vi "23_Roots of Eqn using Case.vi"() -> ()   [LabVIEW 2022 SP3]
panel:
  out "Inference:":string
  out "Root 2":dbl
  out "Root 1":dbl
  in  "C":dbl
  in  "B":dbl
  in  "A":dbl
  # "Develop a HMI to find the roots of an equation and categorize\n whether its Real&Equal or Real&Unequal using Case structure"
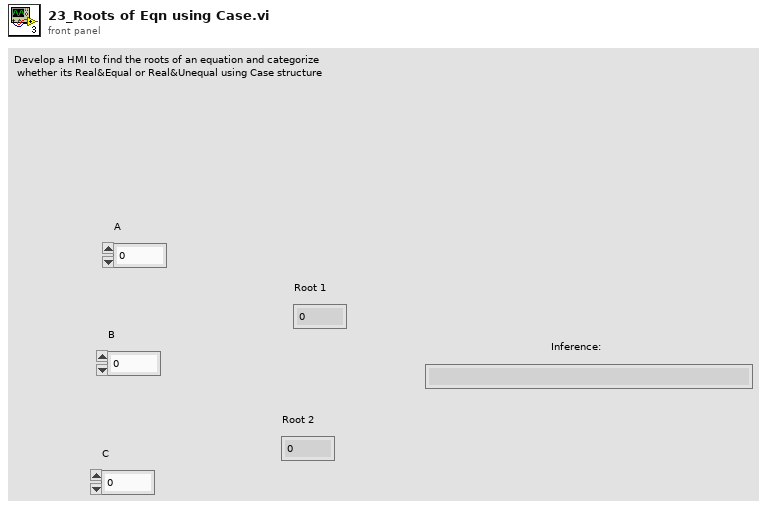
[diagram p1: front panel]
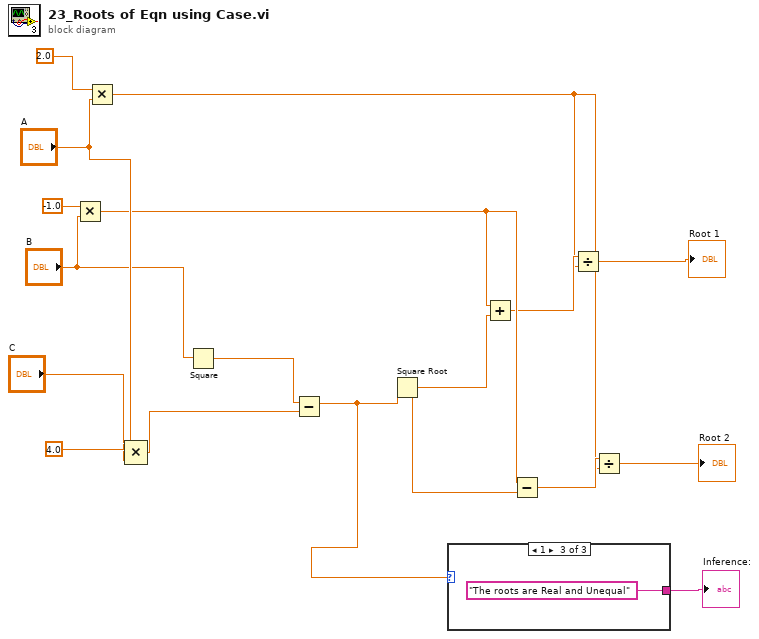
[diagram p0: block diagram]
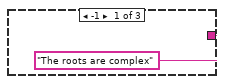
[diagram p2: hidden frame]
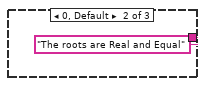
[diagram p3: hidden frame]
diagram:
  n1 = Multiply(x=-1.0, y="B") -> (x*y=w8:dbl)
  n2 = Multiply(x=2.0, y="A") -> (x*y=w5:dbl)
  n3 = Compound Arithmetic op=MULTIPLY(4.0 ("result"), "A", "C") -> (w14:dbl)
  n4 = Square(x="B") -> (x^2=w15:dbl)
  n5 = Subtract(x=w15, y=w14) -> (x-y=w2:dbl)
  n6 = Square Root(x=w2) -> (sqrt(x)=w13:dbl)
  n7 = case shown="1" w2 {
    tunnel: ["The roots are complex" "The roots are Real and Equal" "The roots are Real and Unequal"] -> w1
    frame -1 {
    }
    frame 0, Default {
    }
    frame 1 {
    }
  }
  "Inference:" <- w1
  n8 = Add(x=w8, y=w13) -> (x+y=w7:dbl)
  n9 = Subtract(x=w8, y=w13) -> (x-y=w6:dbl)
  n10 = Divide(x=w7, y=w5) -> (x/y=→"Root 1":dbl)
  n11 = Divide(x=w6, y=w5) -> (x/y=→"Root 2":dbl)
